vi "Ballard XML Generator.Close Channel429.vi"(11 "string in":string) -> (3 "string out":string)   [LabVIEW 2020]
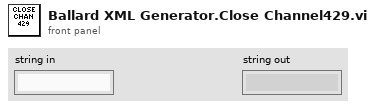
[diagram p1: front panel]
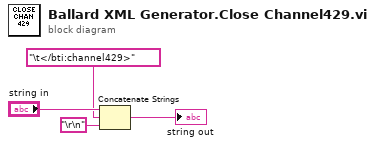
[diagram p0: block diagram]
diagram:
  n1 = Concatenate Strings("string in", "\t</bti:channel429>", "\r\n") -> (→"string out":string)
